vi "Params Globals.vi"() -> ()   [LabVIEW 2010]
panel:
  in  "AxesTypes":enum16{"UE30", "UE72"}[](array[ring])=[enum."UE30", enum."UE72", enum."UE30", enum."UE72"] caption="Type de moteur des axes"
  out "ConvFacts":dbl[](array[numeric])=[1e-06, 1e-05, 0.01, 1e-05] caption="Facteurs de conversion des axes (m/pas ou °/pas)"
  # "W"
  # "W"
  # "X"
  # "X"
  # "Y"
  # "Y"
  # "Z"
  # "Z"
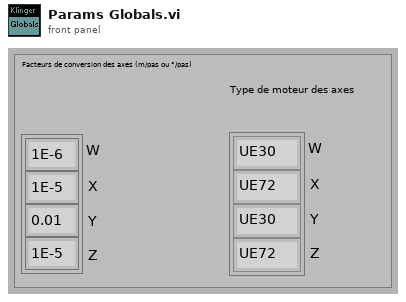
[diagram p1: front panel]
diagram:
